vi "Atheros Xtal Calibration.vi"(6 "error in (no error)":errorcluster, 7 "Parameter In":T1, 9 "_hResourceContext":u32) -> (0 "error out":errorcluster, 2 "function return":bool, 3 "_hResourceContext out":u32)   [LabVIEW 2013, in "QCAWLAN_DLL.lvlib"]
doc: "QCA_DLL_Export bool Atheros_XtalCalibration(HANDLE _hResourceContext, unsigned int channel, int txChainMask, unsigned int gainIndex, int dacGain, int paCfg, unsigned int numAverages);"
uses:
  QCAWLAN_DLL.lvlib
  QCAWLAN_DLL.dll
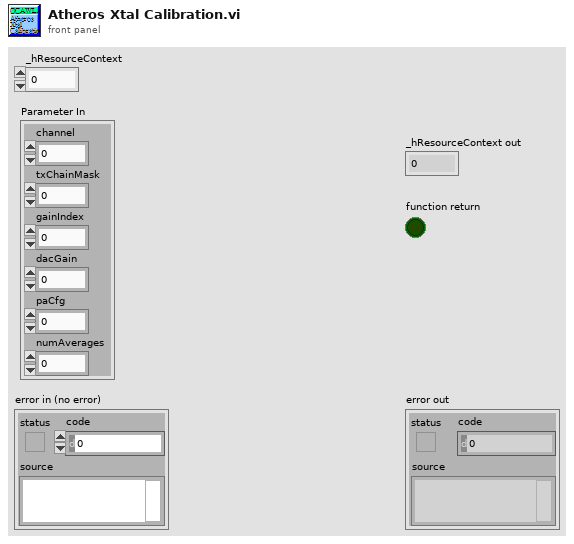
[diagram p1: front panel]
types:
  T1 = cluster{"channel":u32, "txChainMask":i32, "gainIndex":u32, "dacGain":i32, "paCfg":i32, "numAverages":u32}
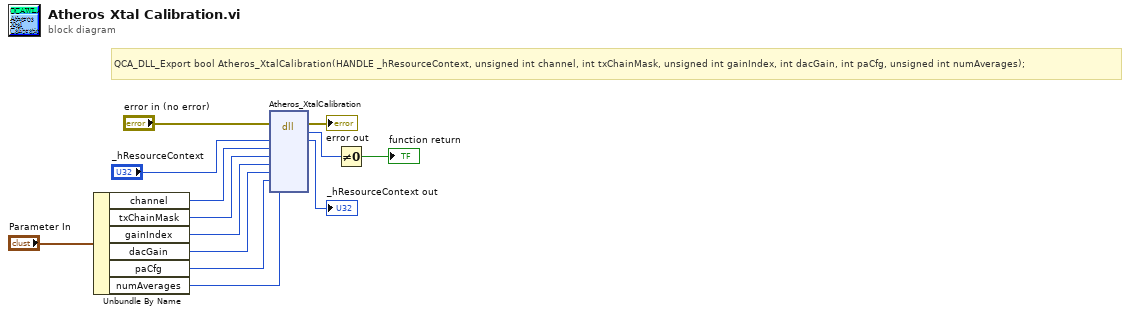
[diagram p0: block diagram]
diagram:
  # "QCA_DLL_Export bool Atheros_XtalCalibration(HANDLE _hResourceContext, unsigned int channel, int txChainMask, unsigned int gainIndex, int dacGain, int paCfg, unsigned int numAverages);"
  n1 = Unbundle By Name("Parameter In") -> ("channel"=w6:u32, "txChainMask"=w5:i32, "gainIndex"=w4:u32, "dacGain"=w3:i32, "paCfg"=w2:i32, "numAverages"=w1:u32)
  n2 = dll-call lib="C:/Connectivity Client - MIMO/PlugIn/QCAWLAN_DLL.*" fn="Atheros_XtalCalibration"(error in="error in (no error)", "_hResourceContext"="_hResourceContext", "channel"=w6, "txChainMask"=w5, "gainIndex"=w4, "dacGain"=w3, "paCfg"=w2, "numAverages"=w1) -> (error out=→"error out":errorcluster, w12:u8, "_hResourceContext"=→"_hResourceContext out":u32)  [unwired: 8 in, 1 out]
  n3 = Not Equal To 0?(x=w12) -> (x != 0?=→"function return":bool)
